vi "setSubnetData.vi"(10 "SubnetData":T1, 11 "Subnet in":refnum<class "ISubnet.lvclass">) -> (3 "Subnet out":refnum<class "ISubnet.lvclass">)   [LabVIEW 2015, in "ISubnet.lvclass"]
uses:
  ISubnet.lvclass
  Subnet/DataTypes/SubnetData.ctl
  Common_RT_Modbus/IModbus/IModbus.lvclass
  Subnet/DataTypes/SubnetConstants.ctl
  Common_RT_HPILC/HPILC/HPILC.lvclass
  Subnet/DataTypes/ILCIndexData.ctl
  Subnet/DataTypes/ILCTypes.ctl
  Subnet/DataTypes/SubnetCommand.ctl
  Subnet/DataTypes/SubnetTelemetry.ctl
  ISubnet.lvclass/ISubnet.ctl
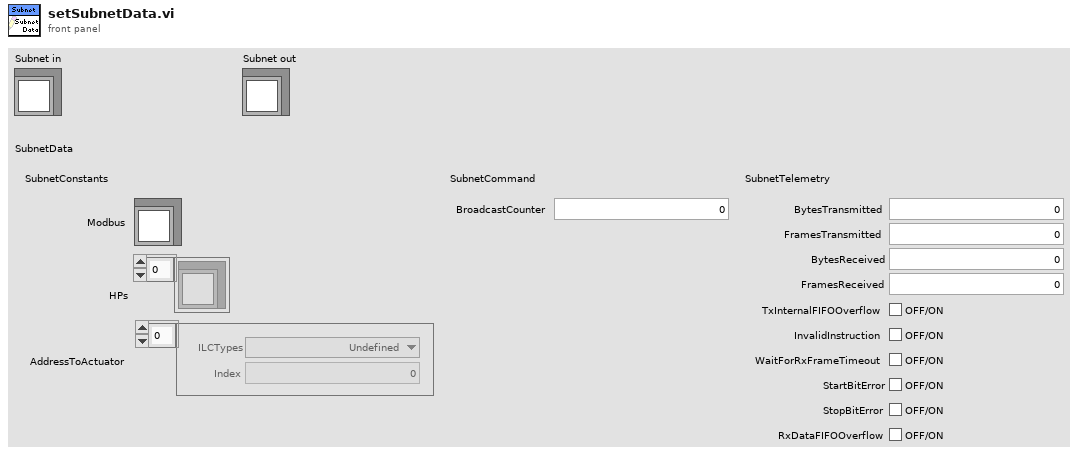
[diagram p1: front panel]
types:
  T1 = typedef "SubnetData.ctl" = cluster{"SubnetConstants":T2, "SubnetCommand":T5, "SubnetTelemetry":T6}
  T2 = typedef "SubnetConstants.ctl" = cluster{"Modbus":refnum<class "IModbus.lvclass">, "HPs":refnum<class "HPILC.lvclass">[], "AddressToActuator":T3[]}
  T3 = typedef "ILCIndexData.ctl" = cluster{"ILCTypes":T4, "Index":i32}
  T4 = typedef "ILCTypes.ctl" = enum16{"Undefined", "SAA", "DAA", "HP"}
  T5 = typedef "SubnetCommand.ctl" = cluster{"BroadcastCounter":u8}
  T6 = typedef "SubnetTelemetry.ctl" = cluster{"BytesTransmitted":u32, "FramesTransmitted":u32, "BytesReceived":u32, "FramesReceived":u32, "TxInternalFIFOOverflow":bool, "InvalidInstruction":bool, "WaitForRxFrameTimeout":bool, "StartBitError":bool, "StopBitError":bool, "RxDataFIFOOverflow":bool}
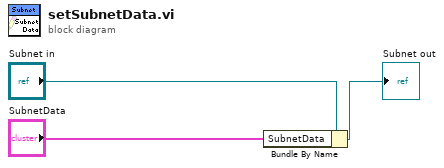
[diagram p0: block diagram]
diagram:
  n1 = Bundle By Name(cluster="Subnet in", "SubnetData"="SubnetData") -> (→"Subnet out":refnum<class "ISubnet.lvclass">)
